vi "Digital Comparison.vi"(0 "Data":bool, 2 "Wait Until":enum8{"Is High", "Is Low"}(ring), 11 "error in":errorcluster) -> (4 "Result":bool, 15 "error out":errorcluster)   [LabVIEW 2010]
doc: "This VI does basic digital comparisons on the Data input."
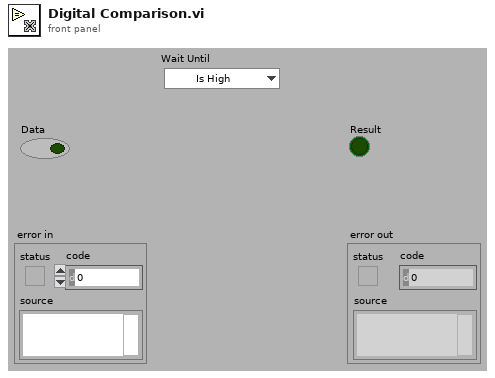
[diagram p1: front panel]
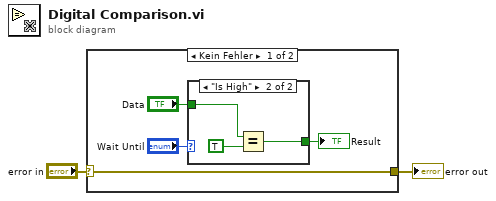
[diagram p0: block diagram]
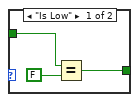
[diagram p2: hidden frame]
diagram:
  n1 = case shown="Kein Fehler" "error in" {
    selector: "error in" -> [w3 w13]
    tunnel: [w3 w13] -> w1
    frame No Error {
      n2 = case shown="\"Is High\"" "Wait Until" {
        tunnel: [w8 w11] -> w5
        tunnel: "Data" -> [w7 w10]
        frame "Is Low" {
          n3 = Equal?(x=w7, y=FALSE) -> (x = y?=w8:bool)
        }
        frame "Is High" {
          n4 = Equal?(x=w10, y=TRUE) -> (x = y?=w11:bool)
        }
      }
      "Result" <- w5
    }
    frame Error {
    }
  }
  "error out" <- w1
